vi "FrameStride.vi"(8 "error in":errorcluster, 11 "camera handle in":u64) -> (0 "error out":errorcluster, 1 "FrameStride (bytes)":i32, 3 "camera handle out":u64)   [LabVIEW 2014, in "PICam.lvlib"]
doc: "Reports the length, in bytes, necessary to traverse to the\nnext frame."
uses:
  PICam.lvlib
  Program Files/Princeton Instruments/PICam/Runtime/Picam32.dll
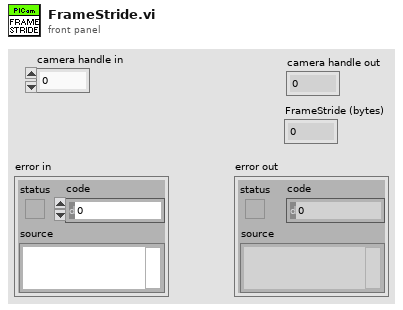
[diagram p1: front panel]
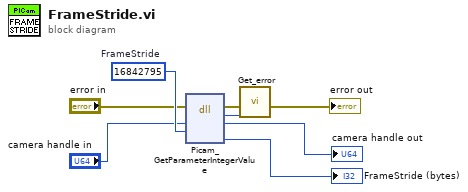
[diagram p0: block diagram]
diagram:
  w4 = u32 16842795  # FrameStride
  n1 = dll-call lib="C:/Program Files/Princeton Instruments/PICam/Runtime/Picam32.dll" fn="Picam_GetParameterIntegerValue"(error in="error in", "camera"="camera handle in", "PicamParameter"=w4) -> (error out=w8:errorcluster, "return type"=w7:i32, "camera"=→"camera handle out":u64, "FrameStride"=→"FrameStride (bytes)":i32)  [unwired: 4 in, 1 out]
  n2 = call "Get_error.vi"("PICam_Error"=w7, "error in (no error)"=w8) -> ("error out"=→"error out":errorcluster)  [unwired: 9 in]
